vi "Add_Stage_Count.vi"(0 "Recipe_Data":string[][](array[string])) -> (4 "Recipe_Data_with_StageCount":string[][](array[string]), 10 "Recipe_Data_Display":string[][](array[string]))   [LabVIEW 2021]
doc: "Used to get the stage count of each recipe."
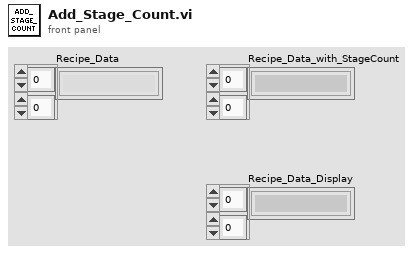
[diagram p1: front panel]
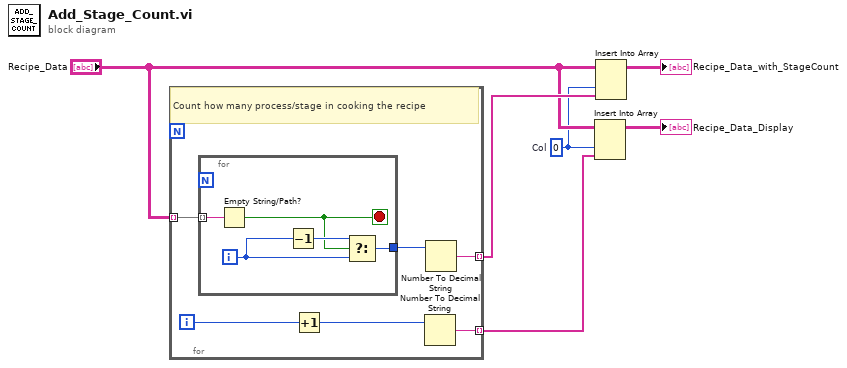
[diagram p0: block diagram]
diagram:
  w1 = 0  # Col
  n1 = for {
    tunnel: "Recipe_Data" -> [w12] mode=indexing
    tunnel: [w10] -> w6 mode=indexing
    tunnel: [w8] -> w3 mode=indexing
    i -> [w9]
    # "Count how many process/stage in cooking the recipe"
    n2 = for {
      tunnel: w12 -> [w17] mode=indexing
      tunnel: [w16] -> w11
      i -> [w15]
      stop <- w13 stop-if-true
      n3 = Empty String/Path?(string/path=w17) -> (empty?=w13:bool)
      n4 = Decrement(x=w15) -> (x-1=w14:i32)
      n5 = Select(t=w14, s=w13, f=w15) -> (s? t:f=w16:i32)
    }
    n6 = Increment(x=w9) -> (x+1=w7:i32)
    n7 = Number To Decimal String(number=w7) -> (decimal integer string=w8:string)  [unwired: 1 in]
    n8 = Number To Decimal String(number=w11) -> (decimal integer string=w10:string)  [unwired: 1 in]
  }
  n9 = Insert Into Array(array="Recipe_Data", index (col)=w1, new element=w3) -> (→"Recipe_Data_Display":string[][])  [unwired: 1 in]
  n10 = Insert Into Array(array="Recipe_Data", index (col)=w1, new element=w6) -> (→"Recipe_Data_with_StageCount":string[][])  [unwired: 1 in]
